vi "Firmware.vi"() -> ()   [LabVIEW 2017]
uses:
  <vilib>/Platform/TimedLoop/XDataNode/timing_clust.ctl
  <vilib>/Platform/TimedLoop/XDataNode/nitl_modes.ctl
  <vilib>/Platform/TimedLoop/XDataNode/wakeup.ctl
  <vilib>/NI/PowerElectronicsControl/Buck-Boost/FPGA/modInput.ctl
  <vilib>/NI/PowerElectronicsControl/ActiveFrontEnd/AFE/Inputs.ctl
  <instrlib>/_niInstr/Instruction Framework/v1/FPGA/Helper Classes/Single Address Space Collection/Single Address Space Collection.lvclass
  C:/Program Files (x86)/National Instruments/LabVIEW 2017/instr.lib/_niInstr/Instruction Framework/v1/FPGA/Interfaces/Address Space Collection/Address Space Collection.lvclass
  <instrlib>/_niInstr/FIFO Register Bus/v1/FPGA/niInstr FIFO Register Bus v1 FPGA.lvclass
  C:/Program Files (x86)/National Instruments/LabVIEW 2017/instr.lib/_niInstr/Instruction Framework/v1/FPGA/Interfaces/Instruction Producer/Instruction Producer.lvclass
  <vilib>/rvi/Emulation/niFpgaGetClockAttributes.vi
  <vilib>/rvi/Emulation/niFpgaSctlEmulationGetInTimedLoop.vi
  <vilib>/rvi/Emulation/niFpgaEmulationReportErrorSimple.vi
  <vilib>/rvi/Emulation/niFpgaProcessEmulError.vi
  <vilib>/rvi/Emulation/niFpgaCriticalErrorInLSC.vi
  <vilib>/rvi/eio/common/nirviEmuTemplateMethod_errors.vi
  <vilib>/rvi/Emulation/niFpgaEmulationIsFPGAContextNoSignature.vi
  <vilib>/rvi/DataTransferAndStorage/Container/Common/niFpgaContainerGetUniqueNameForEmu.vi
  <vilib>/rvi/Memory/Memory_Emulation/niFpgaMemoryEmulationCacheClearOnFirstRun.vi
  <vilib>/rvi/Memory/Memory_Emulation/nirvimemoryEmulationManagerCache_MakeExclusive.vi
  <vilib>/rvi/Memory/Memory_Emulation/niFpgaMemoryEmulationValidateCache.vi
  <vilib>/rvi/Memory/Memory_Emulation/nirvimemoryEmulationManagerCache_InsertValue.vi
  <vilib>/Utility/error.llb/Clear Errors.vi
  <vilib>/rvi/Memory/Memory_Emulation/nirvimemoryEmulationManagerCache_ReleaseExclusive.vi
  <vilib>/rvi/Memory/Memory_Emulation/nirvimemoryEmulationManagerCache_GetValue.vi
  <vilib>/rvi/Memory/Memory_Emulation/nirvimemoryEmulationManagerCache_SetValue.vi
  <userlib>/_NI FLP Library/addons/PowerElectronics/ABCtoAlphaBeta_3PhaseUnitaryMagnitude/FlpLib ABCtoAlphaBeta_3PhaseUnitaryMagnitude 1.vi
  <userlib>/_NI FLP Library/FPGA/outsideSCTL/FlpLib Sine & Cosine Shared Instance 1.vi
  <userlib>/_NI FLP Library/addons/PowerElectronics/AlphaBetaToDQ_noSine/FlpLib AlphaBetaToDQ_noSine 1.vi
  <vilib>/rvi/DataTransferAndStorage/Container/Common/niFpgaContainerExecOnDevCompGetState.vi
  <userlib>/_NI FLP Library/addons/PowerElectronics/SpaceVectorPWM/FlpLib SpaceVectorPWM 2.vi
  <vilib>/rvi/DataTransferAndStorage/Container/Common/niFpgaContainerSetEmuInfo.vi
  <vilib>/rvi/eio/common/nirviEmuReportErrorAndStop.vi
  <vilib>/eio/EIONode/EIONode.xnode
  <vilib>/Platform/TimedLoop/XDataNode/XDataNode.xnode
  <vilib>/rvi/DataTransferAndStorage/Container/XNode/niFpgaContainer.xnode
  <vilib>/rvi/DataTransferAndStorage/Register/Emulation/niFpgaRegisterEmulation.vi
  <vilib>/rvi/DataTransferAndStorage/Register/Emulation/niFpgaRegisterEmulationRefIn.vi
  <vilib>/rvi/LocalResourceManager/LocalResourceManager.xnode
  <instrlib>/_niInstr/Instruction Framework/v1/FPGA/Top Level Bus/Register Configuration/Register Configuration.lvclass
  <vilib>/Platform/TimedLoop/XDataNode/XDNodeRunTimeDep.lvlib
  <vilib>/NI/PowerElectronicsControl/ScaleAndLimit/Core/ScaleAndLimit.lvlib
  <vilib>/NI/PowerElectronicsControl/ScaleAndLimit/Core/AddressSpace.lvclass
  <vilib>/NI/PowerElectronicsControl/WaveformAcq/FPGA/WaveformAddressSpace.lvclass
  <vilib>/NI/PowerElectronicsControl/Buck-Boost/FPGA/BuckBoost.lvlib
  <vilib>/NI/PowerElectronicsControl/Buck-Boost/FPGA/AddressSpace.lvclass
  <vilib>/NI/PowerElectronicsControl/ActiveFrontEnd/AFE/ActiveFrontEnd.lvlib
  <vilib>/NI/PowerElectronicsControl/ActiveFrontEnd/AFE/AddressSpace.lvclass
  <vilib>/NI/PowerElectronicsControl/SVPWM/SVPWM/AddressSpace.lvclass
  <vilib>/NI/PowerElectronicsControl/SVPWM/SVPWM/SVPWM.lvlib
  <vilib>/NI/PowerElectronicsControl/ThreePhasePLL/FPGA/ThreePhasePLL.lvlib
  <vilib>/NI/PowerElectronicsControl/ThreePhasePLL/FPGA/AddressSpace.lvclass
panel:
  out "Vw_AFE":sgl
  out "Vv_AFE":sgl
  out "Vu_AFE":sgl
  out "VLoad":sgl
  out "VDCLink":sgl
  out "gridFrequency":sgl
  in  "PrechargeBuckBoost":bool
  in  "PrechargeAFE":bool
  in  "MainContactor":bool
  in  "ConnectDCLinks":bool
  in  "enableAFE":bool
  in  "I_setpt":sgl format="%#_13g"
  out "I_BuckBoost":sgl[](array[numeric])
  in  "desiredBuckBoostRate":u32
  out "actualBuckBoostRate":u32
  out "FaultBuffer":u64 format="%.0x"
  out "LimitsFlag":bool
  out "Sourcing_P1_DI":u16
  out "Sourcing_P0_DI":u16
  out "Sinking_DO":u32 format="%.0x"
  out "Scanned_AI":sgl[](array[numeric])
  out "AO":i16[](array[numeric])
  out "RelayControl_DO":u8 format="%.0x"
  out "LVTTL_DIO":u32 format="%.0x"
  out "HalfBridge":u16 format="%.0x"
  out "TriggerTimestamp":i32
  out "relativeTimestamp":i32
  in  "ManualTrigger":bool
  in  "fifo reg bus ctrl 0":u32
  out "fifo reg bus status 0":u32
  out "fifo reg bus data 0":u64
  out "SimultaneousAILoopRate":u32
  out "Simultaneous_AI":sgl[](array[numeric])
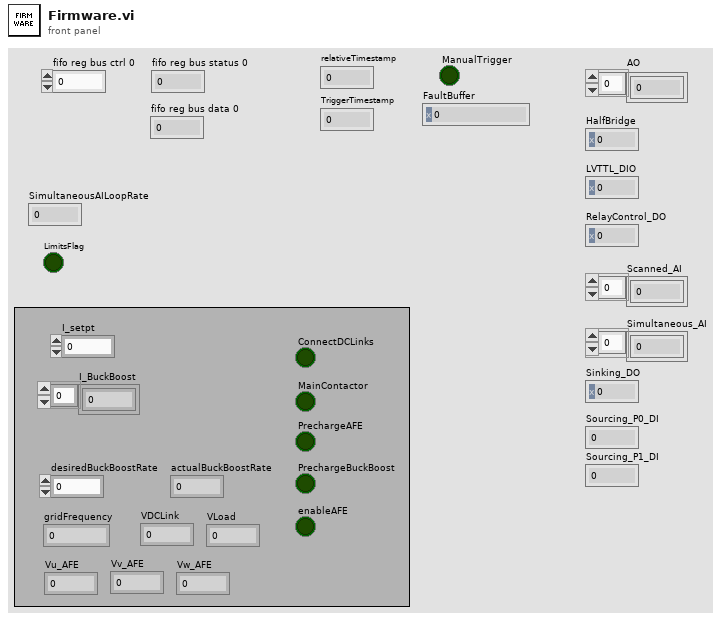
[diagram p1: front panel]
types:
  T1 = typedef "SVPWM.lvlib/Parameters.ctl" = cluster{"Deadtime":refnum<k21>, "Period":refnum<k21>, "A_timing":refnum<k21>, "B_timing":refnum<k21>, "C_timing":refnum<k21>}
  T2 = typedef "BuckBoost.lvlib/contSettings.ctl" = cluster{"numberOfInterleaves":refnum<k21>, "rampRate":refnum<k21>, "manualInput":refnum<k21>, "perturbAmp":refnum<k21>, "perturbAngleInc":refnum<k21>, "reset":refnum<k21>, "state":refnum<k21>, "gains":refnum<k21>, "Currents":refnum<k21>}
  T3 = typedef "BuckBoost.lvlib/modRegisters.ctl" = cluster{"numberOfInterleaves":refnum<k21>, "Enable":refnum<k21>, "triangleInc":refnum<k21>, "Deadband":refnum<k21>, "Enabled":refnum<k21>}
  T4 = typedef "ActiveFrontEnd.lvlib/ControllerRegisters.ctl" = cluster{"Parameters":refnum<k21>, "VDCLinkToP_PISettings":refnum<k21>, "ID_to_VD_PISettings":refnum<k21>, "IQ_to_VQ_PISettings":refnum<k21>, "VDCLink":refnum<k21>, "P":refnum<k21>, "Q":refnum<k21>, "pf":refnum<k21>}
  T5 = typedef "ThreePhasePLL.lvlib/registers.ctl" = cluster{"PLLGains":refnum<k21>, "PLLRange":refnum<k21>, "PLL_reset":refnum<k21>, "PLL_locked":refnum<k21>, "freqBoundaries":refnum<k21>, "expectedFreq":refnum<k21>, "lockDuration":refnum<k21>, "dT":refnum<k21>, "detectedFreq":refnum<k21>, "adjustTheta":refnum<k21>, "HarmonicFilter":refnum<k21>, "HarmonicFilterEnable":refnum<k21>}
  T6 = typedef "XDNodeRunTimeDep.lvlib/timing_clust.ctl" = cluster{"Expected End [f-1]":u64, "Actual End [f-1]":u64, "Finished Late? [f-1]":bool, "Expected End [i-1]":u64, "Actual End [i-1]":u64, "Finished Late? [i-1]":bool, "Expected Start [i]":u64, "Actual Start [i]":u64, "Expected Start [f]":u64, "Actual Start [f]":u64, "Source Name":string, "Structure Name":string, "Period":i64, "Deadline":i64, "Offset":i64, "Start":i64, "Priority":i32, "Timeout":i32, "Mode":T7, "Wakeup Reason":T8, "Error":errorcluster, "Source Type":string, "Secondary Source Type":string, "Global End Time":u64, "Global Start Time":u64, "Frame Duration":u64, "Iteration Duration":u64, "Assigned CPU":i32, "I/O Scan Engine Mode":u32}
  T7 = typedef "XDNodeRunTimeDep.lvlib/nitl_modes.ctl" = enum32{"No Change", "Process missed periods, maintain original phase", "Discard missed periods, maintain original phase", "Process missed periods, ignore original phase", "Discard missed periods, ignore original phase"}
  T8 = typedef "XDNodeRunTimeDep.lvlib/wakeup.ctl" = enum32{"Normal", "Aborted", "Asynchronous wakeup", "Timing source error", "Timed loop error", "Timeout"}
  T9 = typedef "ActiveFrontEnd.lvlib/Inputs.ctl" = cluster{"VgridD":sgl, "VgridQ":sgl, "IgridD":sgl, "IgridQ":sgl, "VDCLink":sgl, "sinTheta":sgl, "cosTheta":sgl}
  T10 = typedef "BuckBoost.lvlib/modInput.ctl" = cluster{"signal":fxp<+,18,0>[]}
  T11 = typedef "niFpgaPID_PIState.ctl" = cluster{"uI(k-1)":sgl, "e(k-1)":sgl, "output (k-1)":sgl}
  T12 = cluster{"PIstateOut":T11, "filter0":sgl, "filter1":sgl}
  T13 = typedef "ActiveFrontEnd.lvlib/Outputs.ctl" = cluster{"VcmdAlpha":sgl, "VcmdBeta":sgl, "VcmdD":sgl, "VcmdQ":sgl, "IcmdD":sgl, "IcmdQ":sgl, "P":sgl, "Q":sgl, "Pf":sgl, "perturbance":sgl}
  T14 = typedef "ON_OFF.ctl" = cluster{"ON":u32, "OFF":u32}
  T15 = typedef "ScaleAndLimit.lvlib/LimitsRegisters.ctl" = cluster{"HighLimits":refnum<k21>, "LowLimits":refnum<k21>, "ClearLimits":refnum<k21>, "LimitsFlag":refnum<k21>}
  T16 = typedef "ScaleAndLimit.lvlib/ConfigRegisters.ctl" = cluster{"LimitsEnabled":refnum<k21>, "UnscaledHighLimit":refnum<k21>, "UnscaledLowLimit":refnum<k21>, "B":refnum<k21>, "M":refnum<k21>}
  T17 = typedef "BuckBoost.lvlib/modOutput.ctl" = cluster{"Top":bool, "Bottom":bool}
  T18 = typedef "SVPWM.lvlib/SwitchPositions.ctl" = cluster{"A_Top":bool, "A_Bot":bool, "B_Top":bool, "B_Bot":bool, "C_Top":bool, "C_Bot":bool}
  T19 = cluster{"VcmdAlpha":sgl, "VcmdBeta":sgl, "VcmdD":sgl, "VcmdQ":sgl, "IcmdD":sgl, "IcmdQ":sgl, "P":sgl, "Q":sgl, "Pf":sgl, "perturbance":sgl}
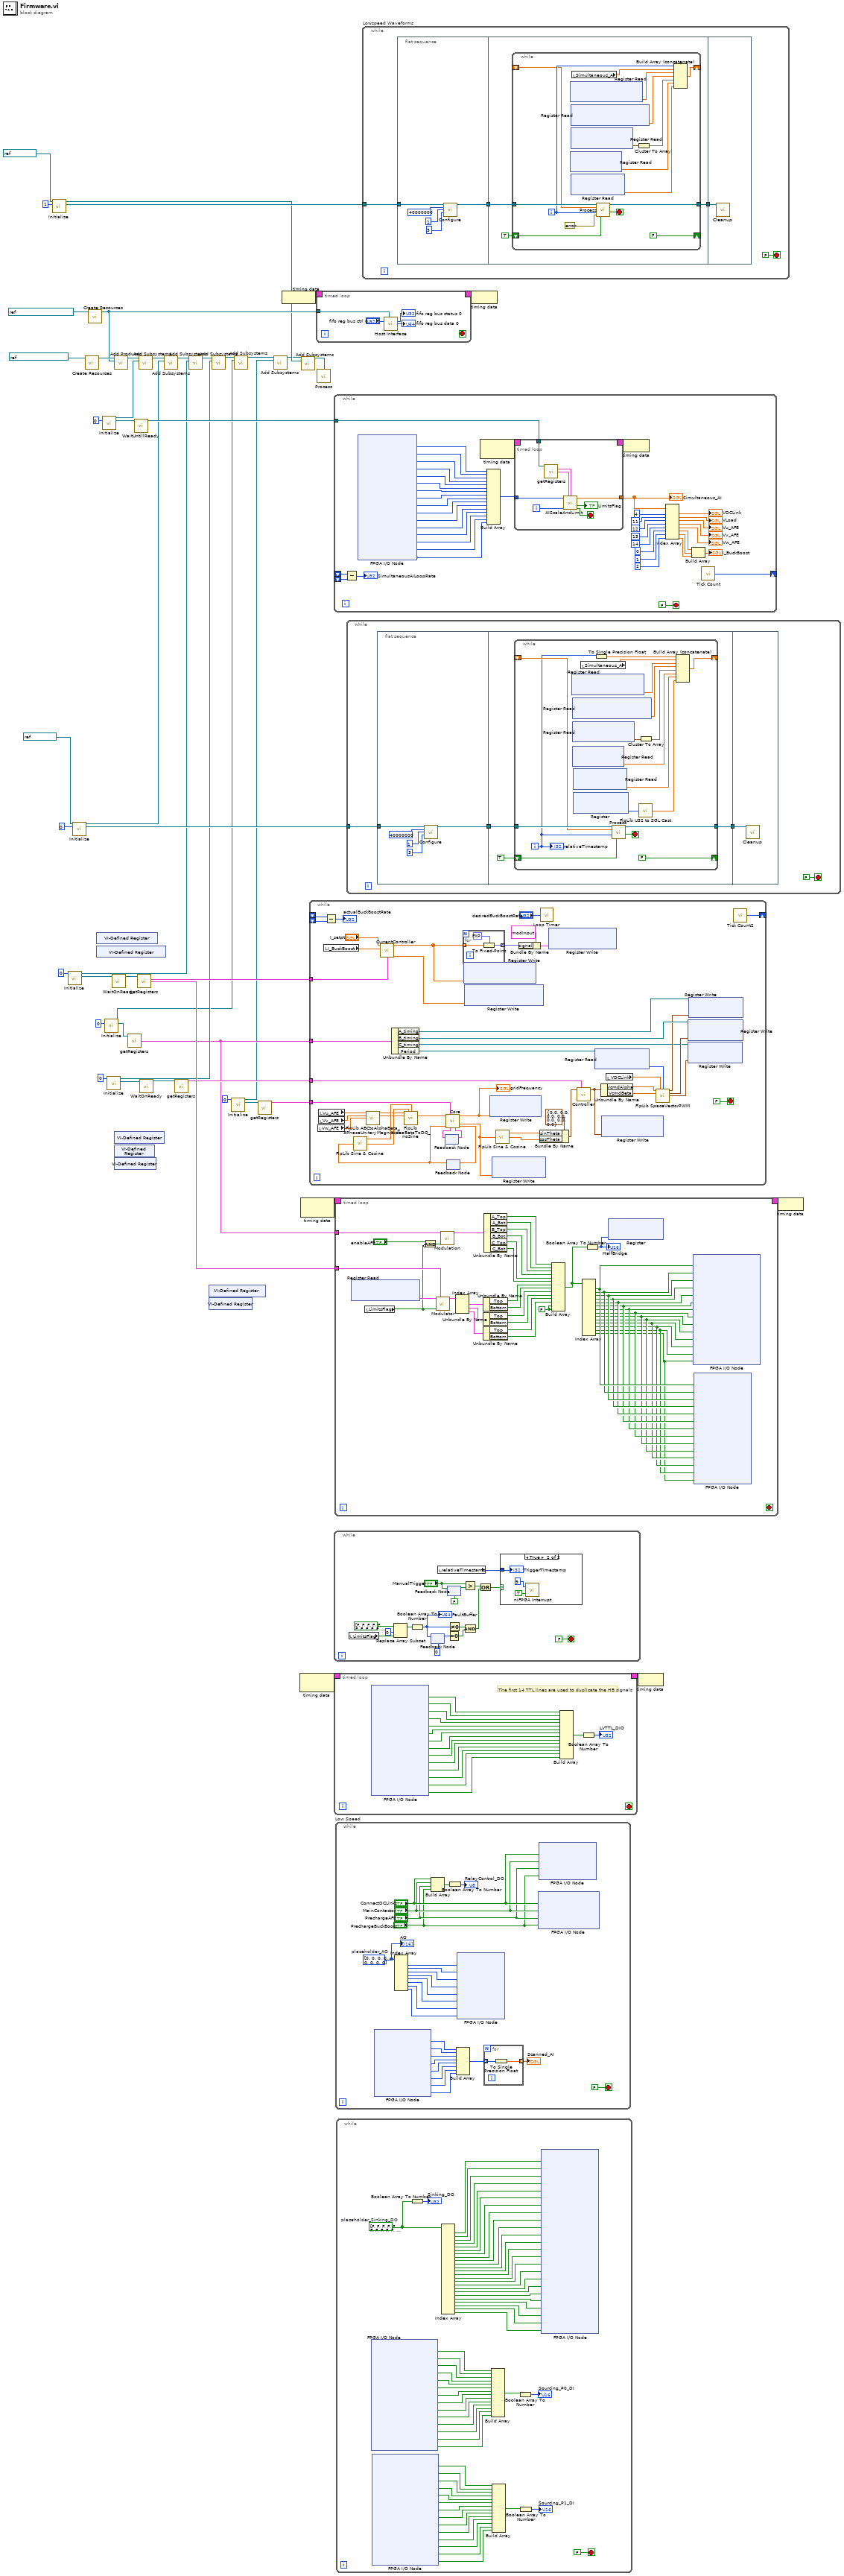
[diagram p0: block diagram]
diagram:
  n1 = call <vilib>:"Initialize.vi"("DMA FIFO"=refnum<k21> "DataSGL1" ("FIFO Out"), "instance"=u8 1) -> ("subsystem"=w28:refnum<class "Single Address Space Collection.lvclass">, "AddressSpace"=w31:refnum<class "WaveformAddressSpace.lvclass">)  [unwired: 12 in]
  n2 = call <vilib>:"Initialize.vi"("instance"=u8 0) -> ("subsystem"=w18:refnum<class "Single Address Space Collection.lvclass">, "AddressSpace"=w24:refnum<class "AddressSpace.lvclass">)  [unwired: 13 in]
  n3 = call <vilib>:"Initialize.vi"("DMA FIFO"=refnum<k21> "DataSGL0" ("FIFO Out"), "instance"=u8 0) -> ("subsystem"=w34:refnum<class "Single Address Space Collection.lvclass">, "AddressSpace"=w36:refnum<class "WaveformAddressSpace.lvclass">)  [unwired: 12 in]
  n4 = call <instrlib>:"Create Resources.vi"("register clock"=refnum<k21> "40 MHz Onboard Clock") -> ("register configuration"=w47:refnum<class "Register Configuration.lvclass">)  [unwired: 14 in]
  n5 = call <instrlib>:"Create Resources.vi"("instruction fifo"=refnum<k21> "reg.host instruction fifo 0") -> ("fifo register bus"=w39:refnum<class "niInstr FIFO Register Bus v1 FPGA.lvclass">)  [unwired: 14 in]
  n6 = xnode "VI-Defined Register"() -> ()  [unwired: 1 out]
  n7 = xnode "VI-Defined Register"() -> ()  [unwired: 1 out]
  n8 = call <vilib>:"Initialize.vi"("instance"=u8 0) -> ("subsystem"=w44:refnum<class "Single Address Space Collection.lvclass">, "AddressSpace"=w42:refnum<class "AddressSpace.lvclass">)  [unwired: 13 in]
  n9 = call <vilib>:"Initialize.vi"("instance"=u8 0) -> ("subsystem"=w8:refnum<class "Single Address Space Collection.lvclass">, "AddressSpace"=w10:refnum<class "AddressSpace.lvclass">)  [unwired: 13 in]
  n10 = call <vilib>:"Initialize.vi"("instance"=u8 0) -> ("subsysytem"=w12:refnum<class "Single Address Space Collection.lvclass">, "AddressSpace"=w16:refnum<class "AddressSpace.lvclass">)  [unwired: 13 in]
  n11 = call <vilib>:"WaitOnReady.vi"("AddressSpace in"=w24) -> ("AddressSpace out"=w23:refnum<class "AddressSpace.lvclass">)  [unwired: 14 in]
  n12 = xnode "VI-Defined Register"() -> ()  [unwired: 1 out]
  n13 = call <instrlib>:"Add Producer.vi"("register configuration in"=w47, "instruction producer"=w39) -> ("register configuration out"=w45:refnum<class "Register Configuration.lvclass">)  [unwired: 13 in]
  n14 = xnode "VI-Defined Register"() -> ()  [unwired: 1 out]
  n15 = xnode "VI-Defined Register"() -> ()  [unwired: 1 out]
  n16 = call <vilib>:"getRegisters.vi"("AddressSpace in"=w10) -> ("Parameters"=w7:T1)  [unwired: 13 in, 1 out]
  n17 = call <vilib>:"WaitUntillReady.vi"("AddressSpace in"=w42) -> ("AddressSpace out"=w41:refnum<class "AddressSpace.lvclass">)  [unwired: 14 in]
  n18 = call <vilib>:"getRegisters.vi"("AddressSpace in"=w23) -> ("settingsReg"=w22:T2, "modRegisters"=w21:T3)  [unwired: 12 in, 1 out]
  n19 = call <instrlib>:"Add Subsystems.vi"("register configuration in"=w45, "subsystems"=w44) -> ("register configuration out"=w35:refnum<class "Register Configuration.lvclass">)  [unwired: 13 in]
  n20 = call <vilib>:"WaitOnReady.vi"("AddressSpace in"=w16) -> ("AddressSpace out"=w15:refnum<class "AddressSpace.lvclass">)  [unwired: 14 in]
  n21 = call <instrlib>:"Add Subsystems.vi"("register configuration in"=w35, "subsystems"=w34) -> ("register configuration out"=w19:refnum<class "Register Configuration.lvclass">)  [unwired: 13 in]
  n22 = call <vilib>:"getRegisters.vi"("AddressSpace in"=w15) -> ("CntlRegisters"=w14:T4)  [unwired: 14 in]
  n23 = call <instrlib>:"Add Subsystems.vi"("register configuration in"=w19, "subsystems"=w18) -> ("register configuration out"=w13:refnum<class "Register Configuration.lvclass">)  [unwired: 13 in]
  n24 = xnode "VI-Defined Register"() -> ()  [unwired: 1 out]
  n25 = xnode "VI-Defined Register"() -> ()  [unwired: 1 out]
  n26 = call <instrlib>:"Add Subsystems.vi"("register configuration in"=w13, "subsystems"=w12) -> ("register configuration out"=w9:refnum<class "Register Configuration.lvclass">)  [unwired: 13 in]
  n27 = call <vilib>:"Initialize.vi"("instance"=u8 0) -> ("subsysytem"=w2:refnum<class "Single Address Space Collection.lvclass">, "AddressSpace"=w6:refnum<class "AddressSpace.lvclass">)  [unwired: 13 in]
  n28 = call <instrlib>:"Add Subsystems.vi"("register configuration in"=w9, "subsystems"=w8) -> ("register configuration out"=w4:refnum<class "Register Configuration.lvclass">)  [unwired: 13 in]
  n29 = call <vilib>:"getRegisters.vi"("AddressSpace"=w6) -> ("registers"=w1:T5)  [unwired: 14 in]
  n30 = call <instrlib>:"Add Subsystems.vi"("register configuration in"=w4, "subsystems"=w2) -> ("register configuration out"=w3:refnum<class "Register Configuration.lvclass">)  [unwired: 13 in]
  n31 = node-c288() -> (w49:T6)
  n32 = node-c288() -> (w33:T6)  [unwired: 1 in]
  n33 = node-c288() -> (w26:T6)  [unwired: 1 in]
  n34 = call <instrlib>:"Add Subsystems.vi"("register configuration in"=w3, "subsystems"=w28) -> ("register configuration out"=w27:refnum<class "Register Configuration.lvclass">)  [unwired: 13 in]
  n35 = while {
    shift-right: [w94] -> _
    shift-left: _ -> [w92]
    shift-left: _ -> [w93]
    tunnel: w22 -> [w89]
    tunnel: w14 -> [w83]
    tunnel: w7 -> [w82]
    tunnel: w1 -> [w66]
    stop <- FALSE stop-if-true
    n36 = local read "Vw_AFE"() -> (w55:sgl)
    n37 = local read "Vu_AFE"() -> (w57:sgl)
    n38 = local read "Vv_AFE"() -> (w56:sgl)
    n39 = local read "I_BuckBoost"() -> (w50:sgl[])
    n40 = Subtract(x=w92, y=w93) -> (x-y=→"actualBuckBoostRate":u32)
    n41 = call-poly <userlib>:"FlpLib ABCtoAlphaBeta_3PhaseUnitaryMagnitude.vi"("A"=w57, "B"=w56, "C"=w55) -> ("alpha"=w68:sgl, "beta"=w69:sgl)  [unwired: 11 in]
    n42 = call <vilib>:"CurrentController.vi"("I_setpt"="I_setpt", "I_procVar"=w50, "settings"=w89) -> ("output"=w60:sgl[], "perturbance"=w59:sgl)  [unwired: 11 in]
    n43 = Unbundle By Name(w82) -> ("A_timing"=w79:refnum<k21>, "B_timing"=w78:refnum<k21>, "C_timing"=w75:refnum<k21>, "Period"=w81:refnum<k21>)
    n44 = feedback #1() -> (w51:T12)  [unwired: 1 in]
    n45 = feedback #2() -> (w73:sgl)  [unwired: 1 in]
    n46 = call-poly <userlib>:"FlpLib Sine & Cosine.vi"("x"=w73) -> ("cos(x)"=w70:sgl, "sin(x)"=w71:sgl)  [unwired: 3 in]
    n47 = call-poly <userlib>:"FlpLib AlphaBetaToDQ_noSine.vi"("alpha"=w68, "cosx"=w70, "sinx"=w71, "beta"=w69) -> ("quadrature"=w72:sgl)  [unwired: 10 in, 1 out]
    n48 = call <vilib>:"Core.vi"("Vq"=w72, "registers"=w66, "ThetaIn"=w73, "StateIn"=w51) -> ("gridFrequency"=w54:sgl, "adjustedTheta"=w53:sgl, "StateOut"=w52:T12, "ThetaOut"=w67:sgl)  [unwired: 7 in, 1 out]
    "gridFrequency" <- w54
    n49 = feedback-in #1(w52) -> ()
    n50 = feedback-in #2(w67) -> ()
    n51 = for {
      tunnel: w60 -> [w97] mode=indexing
      tunnel: [w98] -> w87 mode=indexing
      n52 = To Fixed-Point(fixed-point type=fxp<+,18,0> 0.0 ("triangle"), number=w97) -> (fixed-point=w98:fxp<+,18,0>)
    }
    n53 = xnode ("Register Write")("Data"=w60) -> ()  [unwired: 1 in, 1 out]
    n54 = xnode ("Register Write")("Data"=w59) -> ()  [unwired: 1 in, 1 out]
    n55 = xnode ("Register Write")("Data"=w54) -> ()  [unwired: 1 in, 1 out]
    n56 = xnode ("Register Write")("Data"=w53) -> ()  [unwired: 1 in, 1 out]
    n57 = call-poly <userlib>:"FlpLib Sine & Cosine.vi"("x"=w53) -> ("cos(x)"=w63:sgl, "sin(x)"=w64:sgl)  [unwired: 3 in]
    n58 = Bundle By Name(cluster=T10 {"signal"=[0.0, 0.0, 0.0, 0.0]} ("input"), "signal"=w87) -> (w86:T10)
    n59 = Bundle By Name(cluster=T9 {"VgridD"=0.0, "VgridQ"=0.0, "IgridD"=0.0, "IgridQ"=0.0, "VDCLink"=0.0, "sinTheta"=0.0, "cosTheta"=0.0} ("Inputs"), "sinTheta"=w64, "cosTheta"=w63) -> (w62:T9)
    n60 = call "Loop Timer"("Count(Ticks)"="desiredBuckBoostRate") -> ()  [unwired: 1 out]
    n61 = xnode ("Register Write")("Data"=w86) -> ()  [unwired: 1 in, 1 out]
    n62 = call <vilib>:"Controller.vi"("Inputs"=w62, "Registers"=w83) -> ("Outputs"=w61:T13)  [unwired: 13 in]
    n63 = xnode ("Register Read")("Register In"=w81) -> ("Data"=w80:u32)  [unwired: 1 out]
    n64 = Unbundle By Name(w61) -> ("VcmdAlpha"=w84:sgl, "VcmdBeta"=w85:sgl)
    n65 = xnode ("Register Write")("Data"=w61) -> ()  [unwired: 1 in, 1 out]
    n66 = local read "VDCLink"() -> (w58:sgl)
    n67 = call-poly <userlib>:"FlpLib SpaceVectorPWM.vi"("ref_alpha"=w84, "ref_max"=w58, "Period"=w80, "ref_beta"=w85) -> ("A"=w77:T14, "B"=w76:T14, "C"=w74:T14)  [unwired: 8 in, 1 out]
    n68 = xnode ("Register Write")("Data"=w74, "Register In"=w75) -> ()  [unwired: 1 out]
    n69 = xnode ("Register Write")("Data"=w76, "Register In"=w78) -> ()  [unwired: 1 out]
    n70 = xnode ("Register Write")("Data"=w77, "Register In"=w79) -> ()  [unwired: 1 out]
    n71 = call "Tick Count2"() -> ("Tick Count(Ticks)"=w94:u32)
  }
  n72 = timed-loop {
    timing: w49 -> [_]
    timing-out: [_] -> w48
    tunnel: w39 -> [w103]
    stop <- _ stop-if-true
    n73 = call <instrlib>:"Host Interface.vi"("fifo register bus"=w103, "fifo reg bus ctrl 0"="fifo reg bus ctrl 0") -> ("fifo reg bus status 0"=→"fifo reg bus status 0":u32, "fifo reg bus data 0"=→"fifo reg bus data 0":u64)  [unwired: 12 in]
  }
  n74 = call <instrlib>:"Process.vi"("register configuration"=w27) -> ()  [unwired: 15 in]
  n75 = while {
    shift-right: [w147] -> _
    shift-left: _ -> [w146]
    shift-left: _ -> [w145]
    tunnel: w41 -> [w135]
    stop <- FALSE stop-if-true
    n76 = Subtract(x=w146, y=w145) -> (x-y=→"SimultaneousAILoopRate":u32)
    n77 = xnode "FPGA I/O Node"() -> ("I0_BuckBoost"=w143:i16, "I1_BuckBoost"=w142:i16, "I2_BuckBoost"=w141:i16, "Vgrid_BuckBoost"=w140:i16, "VDCLink_BuckBoost"=w139:i16, "V0_BuckBoost"=w138:i16, "V1_BuckBoost"=w133:i16, "V2_BuckBoost"=w132:i16, "Iu_AFE"=w131:i16, "Iv_AFE"=w130:i16, "Iw_AFE"=w129:i16, "VLoad_BuckBoost"=w128:i16, "Vu_AFE"=w127:i16, "Vv_AFE"=w126:i16, "Vw_AFE"=w125:i16, "VDCLink_AFE"=w124:i16)  [unwired: 16 in, 16 out]
    n78 = node-c288() -> (w137:T6)  [unwired: 1 in]
    n79 = Build Array(w143, w142, w141, w140, w139, w138, w133, w132, w131, w130, w129, w128, w127, w126, w125, w124) -> (w134:i16[])
    n80 = timed-loop {
      timing: w137 -> [_]
      timing-out: [_] -> w136
      tunnel: w134 -> [w156]
      tunnel: [w155] -> w123
      tunnel: w135 -> [w153]
      i -> [w150]
      stop <- w154 stop-if-true
      n81 = call <vilib>:"getRegisters.vi"("AddressSpace in"=w153) -> ("LimitsRegisters"=w151:T15, "ConfigRegisters"=w152:T16)  [unwired: 12 in, 1 out]
      n82 = call <vilib>:"AIScaleAndLimit.vi"("UnscaledAI"=w156, "ConfigRegisters"=w152, "LimitsRegisters"=w151, "index"=w150) -> ("ScaledAI"=w155:sgl[], "Limited"=→"LimitsFlag":bool, "output valid"=w154:bool)  [unwired: 9 in]
    }
    "Simultaneous_AI" <- w123
    n83 = node-c288(w136) -> ()
    n84 = Index Array(array=w123, index #1=4 ("index"), index #2=11 ("index"), index #3=12 ("index"), index #4=13 ("index"), index #5=14 ("index"), index #6=0 ("index"), index #7=1 ("index"), index #8=2 ("index")) -> (element #1=→"VDCLink":sgl, element #2=→"VLoad":sgl, element #3=→"Vu_AFE":sgl, element #4=→"Vv_AFE":sgl, element #5=→"Vw_AFE":sgl, element #6=w109:sgl, element #7=w108:sgl, element #8=w107:sgl)
    n85 = Build Array(w109, w108, w107) -> (→"I_BuckBoost":sgl[])
    n86 = call "Tick Count"() -> ("Tick Count(Ticks)"=w147:u32)
  }
  n87 = while {
    stop <- FALSE stop-if-true
    n88 = local read "LimitsFlag"() -> (w169:bool)
    n89 = Replace Array Subset(array=bool[] [FALSE, FALSE, FALSE, FALSE, FALSE, FALSE, FALSE, FALSE, FALSE, FALSE, FALSE, FALSE, FALSE, FALSE, FALSE, FALSE, FALSE, FALSE, FALSE, FALSE, FALSE, FALSE, FALSE, FALSE, FALSE, FALSE, FALSE, FALSE, FALSE, FALSE, FALSE, FALSE, FALSE, FALSE, FALSE, FALSE, FALSE, FALSE, FALSE, FALSE, FALSE, FALSE, FALSE, FALSE, FALSE, FALSE, FALSE, FALSE, FALSE, FALSE, FALSE, FALSE, FALSE, FALSE, FALSE, FALSE, FALSE, FALSE, FALSE, FALSE, FALSE, FALSE, FALSE, FALSE], new element=w169, index=0) -> (w167:bool[])
    n90 = Boolean Array To Number(Boolean array=w167) -> (number=w165:u64)
    "FaultBuffer" <- w165
    n91 = feedback-in #3(w165) -> ()
    n92 = feedback #3(u64 0) -> (w164:u64)
    n93 = local read "relativeTimestamp"() -> (w171:i32)
    n94 = feedback-in #4("ManualTrigger") -> ()
    n95 = feedback #4(FALSE ("ManualTrigger")) -> (w175:bool)
    n96 = Equal To 0?(x=w164) -> (x = 0?=w162:bool)
    n97 = Not Equal To 0?(x=w165) -> (x != 0?=w163:bool)
    n98 = Greater?(x="ManualTrigger", y=w175) -> (0:w176:bool)
    n99 = Compound Arithmetic op=AND(w163, w162) -> (w161:bool)
    n100 = Compound Arithmetic op=OR(w176, w161) -> (w173:bool)
    n101 = case shown="True" w173 {
      tunnel: w171 -> [_ w178]
      frame False {
      }
      frame True {
        n102 = call <vilib>:"niFPGA Interrupt.vi"("Wait Until Cleared (F)"=TRUE, "IRQ Number (0)"=u8 9) -> ()  [unwired: 1 in]
        "TriggerTimestamp" <- w178
      }
    }
  }
  n103 = timed-loop {
    timing: w33 -> [_]
    timing-out: [_] -> w32
    stop <- _ stop-if-true
    # "The first 14 TTL lines are used to duplicate the HB signals"
    n104 = xnode "FPGA I/O Node"() -> ("RMC/LVTTL/DIO18"=w196:bool, "RMC/LVTTL/DIO19"=w195:bool, "RMC/LVTTL/DIO20"=w194:bool, "RMC/LVTTL/DIO21"=w193:bool, "RMC/LVTTL/DIO22"=w192:bool, "RMC/LVTTL/DIO23"=w191:bool, "RMC/LVTTL/DIO24"=w190:bool, "RMC/LVTTL/DIO25"=w189:bool, "RMC/LVTTL/DIO26"=w188:bool, "RMC/LVTTL/DIO27"=w187:bool, "RMC/LVTTL/DIO28"=w186:bool, "RMC/LVTTL/DIO29"=w185:bool, "RMC/LVTTL/DIO30"=w184:bool, "RMC/LVTTL/DIO31"=w183:bool)  [unwired: 14 in, 14 out]
    n105 = Build Array(w196, w195, w194, w193, w192, w191, w190, w189, w188, w187, w186, w185, w184, w183) -> (w182:bool[])
    n106 = Boolean Array To Number(Boolean array=w182) -> (number=→"LVTTL_DIO":u16)
  }
  n107 = timed-loop {
    timing: w26 -> [_]
    timing-out: [_] -> w25
    tunnel: w21 -> [w238]
    tunnel: w7 -> [w236]
    stop <- _ stop-if-true
    w200 = FALSE ("element")
    n108 = xnode ("Register Read")() -> ("Data"=w237:cluster{"signal":fxp<+,18,0>[]})  [unwired: 1 in, 1 out]
    n109 = local read "LimitsFlag"() -> (w234:bool)
    n110 = Compound Arithmetic op=AND("enableAFE", invert w234) -> (w233:bool)
    n111 = call <vilib>:"Modulator.vi"("input"=w237, "modRegisters"=w238, "Disable"=w234) -> ("output"=w232:T17[])  [unwired: 12 in]
    n112 = call <vilib>:"Modulation.vi"("Parameters"=w236, "enable"=w233) -> ("SwitchPositions"=w228:T18)  [unwired: 13 in]
    n113 = Index Array(array=w232) -> (element #1=w231:T17, element #2=w230:T17, element #3=w229:T17)  [unwired: 3 in]
    n114 = Unbundle By Name(w231) -> ("Top"=w221:bool, "Bottom"=w220:bool)
    n115 = Unbundle By Name(w230) -> ("Top"=w219:bool, "Bottom"=w218:bool)
    n116 = Unbundle By Name(w229) -> ("Top"=w217:bool, "Bottom"=w216:bool)
    n117 = Unbundle By Name(w228) -> ("A_Top"=w227:bool, "A_Bot"=w226:bool, "B_Top"=w225:bool, "B_Bot"=w224:bool, "C_Top"=w223:bool, "C_Bot"=w222:bool)
    n118 = Build Array(w227, w226, w225, w224, w223, w222, w221, w220, w219, w218, w217, w216, w200, w200) -> (w215:bool[])
    n119 = Index Array(array=w215) -> (element #1=w214:bool, element #2=w213:bool, element #3=w212:bool, element #4=w211:bool, element #5=w210:bool, element #6=w209:bool, element #7=w208:bool, element #8=w207:bool, element #9=w206:bool, element #10=w205:bool, element #11=w204:bool, element #12=w203:bool, element #13=w202:bool, element #14=w201:bool)  [unwired: 14 in]
    n120 = Boolean Array To Number(Boolean array=w215) -> (number=w199:u16)
    "HalfBridge" <- w199
    n121 = xnode "Register"("Data"=w199) -> ()  [unwired: 1 in, 1 out]
    n122 = xnode "FPGA I/O Node"("RMC/Half-Bridge/DO0"=w214, "RMC/Half-Bridge/DO1"=w213, "RMC/Half-Bridge/DO2"=w212, "RMC/Half-Bridge/DO3"=w211, "RMC/Half-Bridge/DO4"=w210, "RMC/Half-Bridge/DO5"=w209, "RMC/Half-Bridge/DO6"=w208, "RMC/Half-Bridge/DO7"=w207, "RMC/Half-Bridge/DO8"=w206, "RMC/Half-Bridge/DO9"=w205, "RMC/Half-Bridge/DO10"=w204, "RMC/Half-Bridge/DO11"=w203, "RMC/Half-Bridge/DO12"=w202, "RMC/Half-Bridge/DO13"=w201) -> ()  [unwired: 14 in, 14 out]
    n123 = xnode "FPGA I/O Node"("RMC/LVTTL/DIO0"=w214, "RMC/LVTTL/DIO1"=w213, "RMC/LVTTL/DIO2"=w212, "RMC/LVTTL/DIO3"=w211, "RMC/LVTTL/DIO4"=w210, "RMC/LVTTL/DIO5"=w209, "RMC/LVTTL/DIO6"=w208, "RMC/LVTTL/DIO7"=w207, "RMC/LVTTL/DIO8"=w206, "RMC/LVTTL/DIO9"=w205, "RMC/LVTTL/DIO10"=w204, "RMC/LVTTL/DIO11"=w203, "RMC/LVTTL/DIO12"=w202, "RMC/LVTTL/DIO13"=w201) -> ()  [unwired: 14 in, 14 out]
  }
  n124 = while "Low Speed" {
    stop <- FALSE stop-if-true
    w265 = i16[] [0, 0, 0, 0, 0, 0, 0, 0]  # placeholder_AO
    n125 = xnode "FPGA I/O Node"() -> ("RMC/Scanned/AI0"=w255:i16, "RMC/Scanned/AI1"=w254:i16, "RMC/Scanned/AI2"=w253:i16, "RMC/Scanned/AI3"=w252:i16, "RMC/Scanned/AI4"=w251:i16, "RMC/Scanned/AI5"=w250:i16, "RMC/Scanned/AI6"=w249:i16, "RMC/Scanned/AI7"=w248:i16)  [unwired: 8 in, 8 out]
    n126 = Index Array(array=w265) -> (element #1=w264:i16, element #2=w263:i16, element #3=w262:i16, element #4=w261:i16, element #5=w260:i16, element #6=w259:i16, element #7=w258:i16, element #8=w257:i16)  [unwired: 8 in]
    n127 = Build Array("ConnectDCLinks", "MainContactor", "PrechargeAFE", "PrechargeBuckBoost") -> (w245:bool[])
    n128 = Boolean Array To Number(Boolean array=w245) -> (number=→"RelayControl_DO":u8)
    n129 = Build Array(w255, w254, w253, w252, w251, w250, w249, w248) -> (w247:i16[])
    n130 = xnode "FPGA I/O Node"("RMC/AO/AO0"=w264, "RMC/AO/AO1"=w263, "RMC/AO/AO2"=w262, "RMC/AO/AO3"=w261, "RMC/AO/AO4"=w260, "RMC/AO/AO5"=w259, "RMC/AO/AO6"=w258, "RMC/AO/AO7"=w257) -> ()  [unwired: 8 in, 8 out]
    n131 = for {
      tunnel: w247 -> [w268] mode=indexing
      tunnel: [w267] -> w246 mode=indexing
      n132 = To Single Precision Float(number=w268) -> (single precision float=w267:sgl)
    }
    "Scanned_AI" <- w246
    n133 = xnode "FPGA I/O Node"("ConnectDCLinks"="ConnectDCLinks", "MainContactor"="MainContactor", "PrechargeAFE"="PrechargeAFE", "PrechargeBuckBoost"="PrechargeBuckBoost") -> ()  [unwired: 4 in, 4 out]
    n134 = xnode "FPGA I/O Node"("RMC/LVTTL/DIO14"="ConnectDCLinks", "RMC/LVTTL/DIO15"="MainContactor", "RMC/LVTTL/DIO16"="PrechargeAFE", "RMC/LVTTL/DIO17"="PrechargeBuckBoost") -> ()  [unwired: 4 in, 4 out]
    "AO" <- w265
  }
  n135 = while {
    stop <- FALSE stop-if-true
    w326 = bool[] [FALSE, FALSE, FALSE, FALSE, FALSE, FALSE, FALSE, FALSE, FALSE, FALSE, FALSE, FALSE, FALSE, FALSE, FALSE, FALSE, FALSE, FALSE, FALSE, FALSE, FALSE, FALSE, FALSE, FALSE]  # placeholder_Sinking_DO
    n136 = xnode "FPGA I/O Node"() -> ("RMC/Sourcing P0/DI0"=w300:bool, "RMC/Sourcing P0/DI1"=w299:bool, "RMC/Sourcing P0/DI2"=w298:bool, "RMC/Sourcing P0/DI3"=w297:bool, "RMC/Sourcing P0/DI4"=w296:bool, "RMC/Sourcing P0/DI5"=w295:bool, "RMC/Sourcing P0/DI6"=w294:bool, "RMC/Sourcing P0/DI7"=w293:bool, "RMC/Sourcing P0/DI8"=w292:bool, "RMC/Sourcing P0/DI9"=w291:bool, "RMC/Sourcing P0/DI10"=w290:bool, "RMC/Sourcing P0/DI11"=w289:bool, "RMC/Sourcing P0/DI12"=w288:bool, "RMC/Sourcing P0/DI13"=w287:bool)  [unwired: 14 in, 14 out]
    n137 = xnode "FPGA I/O Node"() -> ("RMC/Sourcing P1/DI0"=w269:bool, "RMC/Sourcing P1/DI1"=w270:bool, "RMC/Sourcing P1/DI2"=w271:bool, "RMC/Sourcing P1/DI3"=w272:bool, "RMC/Sourcing P1/DI4"=w273:bool, "RMC/Sourcing P1/DI5"=w274:bool, "RMC/Sourcing P1/DI6"=w275:bool, "RMC/Sourcing P1/DI7"=w276:bool, "RMC/Sourcing P1/DI8"=w277:bool, "RMC/Sourcing P1/DI9"=w278:bool, "RMC/Sourcing P1/DI10"=w279:bool, "RMC/Sourcing P1/DI11"=w280:bool, "RMC/Sourcing P1/DI12"=w281:bool, "RMC/Sourcing P1/DI13"=w282:bool)  [unwired: 14 in, 14 out]
    n138 = Boolean Array To Number(Boolean array=w326) -> (number=→"Sinking_DO":u32)
    n139 = Index Array(array=w326) -> (element #1=w325:bool, element #2=w324:bool, element #3=w323:bool, element #4=w322:bool, element #5=w321:bool, element #6=w320:bool, element #7=w319:bool, element #8=w318:bool, element #9=w317:bool, element #10=w316:bool, element #11=w315:bool, element #12=w314:bool, element #13=w313:bool, element #14=w312:bool, element #15=w311:bool, element #16=w310:bool, element #17=w309:bool, element #18=w308:bool, element #19=w307:bool, element #20=w306:bool, element #21=w305:bool, element #22=w304:bool, element #23=w303:bool, element #24=w302:bool)  [unwired: 24 in]
    n140 = Build Array(w300, w299, w298, w297, w296, w295, w294, w293, w292, w291, w290, w289, w288, w287) -> (w286:bool[])
    n141 = Build Array(w269, w270, w271, w272, w273, w274, w275, w276, w277, w278, w279, w280, w281, w282) -> (w283:bool[])
    n142 = Boolean Array To Number(Boolean array=w286) -> (number=→"Sourcing_P0_DI":u16)
    n143 = Boolean Array To Number(Boolean array=w283) -> (number=→"Sourcing_P1_DI":u16)
    n144 = xnode "FPGA I/O Node"("RMC/Sinking/DO0"=w325, "RMC/Sinking/DO1"=w324, "RMC/Sinking/DO2"=w323, "RMC/Sinking/DO3"=w322, "RMC/Sinking/DO4"=w321, "RMC/Sinking/DO5"=w320, "RMC/Sinking/DO6"=w319, "RMC/Sinking/DO7"=w318, "RMC/Sinking/DO8"=w317, "RMC/Sinking/DO9"=w316, "RMC/Sinking/DO10"=w315, "RMC/Sinking/DO11"=w314, "RMC/Sinking/DO12"=w313, "RMC/Sinking/DO13"=w312, "RMC/Sinking/DO14"=w311, "RMC/Sinking/DO15"=w310, "RMC/Sinking/DO16"=w309, "RMC/Sinking/DO17"=w308, "RMC/Sinking/DO18"=w307, "RMC/Sinking/DO19"=w306, "RMC/Sinking/DO20"=w305, "RMC/Sinking/DO21"=w304, "RMC/Sinking/DO22"=w303, "RMC/Sinking/DO23"=w302) -> ()  [unwired: 24 in, 24 out]
  }
  n145 = while {
    tunnel: w36 -> [w328]
    stop <- FALSE stop-if-true
    n146 = flat-sequence {
      tunnel: [w332] -> w330
      tunnel: w328 -> [w333]
      tunnel: w330 -> [w339]
      tunnel: [w338] -> w329
      tunnel: w329 -> [w358]
      frame #0 {
        n147 = call <vilib>:"Configure.vi"("WaveformAddressSpace in"=w333, "oclk_freq"=u32 40000000, "oclk_mult"=u32 1, "UnderflowMargin"=u32 3 ("y")) -> ("WaveformAddressSpace out"=w332:refnum<class "WaveformAddressSpace.lvclass">)  [unwired: 11 in]
      }
      frame #1 {
        n148 = while {
          shift-right: [w356] -> _
          shift-left: _ -> [w350]
          shift-right: [FALSE] -> _
          shift-left: TRUE -> [w352]
          tunnel: w339 -> [w354]
          tunnel: [w353] -> w338
          i -> [w349]
          stop <- w355 stop-if-true
          n149 = xnode ("Register Read")() -> ("Data"=w346:sgl[])  [unwired: 1 in, 1 out]
          n150 = xnode ("Register Read")() -> ("Data"=w345:sgl)  [unwired: 1 in, 1 out]
          n151 = xnode ("Register Read")() -> ("Data"=w347:T19)  [unwired: 1 in, 1 out]
          n152 = xnode ("Register Read")() -> ("Data"=w343:sgl)  [unwired: 1 in, 1 out]
          n153 = xnode "Register"() -> ("Data"=w341:u16)  [unwired: 1 in, 1 out]
          n154 = xnode ("Register Read")() -> ("Data"=w342:sgl)  [unwired: 1 in, 1 out]
          n155 = local read "Simultaneous_AI"() -> (w351:sgl[])
          n156 = To Single Precision Float(number=w349) -> (single precision float=w348:sgl)
          n157 = call <instrlib>:"Process.vi"("WaveformAddressSpace in"=w354, "Data"=w350, "Iteration"=w349, "FirstIteration"=w352) -> ("WaveformAddressSpace out"=w353:refnum<class "WaveformAddressSpace.lvclass">, "stop"=w355:bool)  [unwired: 8 in, 2 out]
          n158 = call <userlib>:"FlpLib U32 to SGL Cast.vi"("x"=w341) -> ("y"=w340:sgl)  [unwired: 4 in]
          n159 = Cluster To Array(cluster=w347) -> (array=w344:sgl[])
          n160 = Build Array (concatenate)(w348, w351, w346, w345, w344, w343, w342, w340) -> (w356:sgl[])
          "relativeTimestamp" <- w349
        }
      }
      frame #2 {
        n161 = call <vilib>:"Cleanup.vi"("WaveformAddressSpace in"=w358) -> ()  [unwired: 14 in, 1 out]
      }
    }
  }
  n162 = while "Lowspeed Waveforms" {
    tunnel: w31 -> [w359]
    stop <- FALSE stop-if-true
    n163 = flat-sequence {
      tunnel: [w363] -> w361
      tunnel: w359 -> [w364]
      tunnel: w361 -> [w370]
      tunnel: [w369] -> w360
      tunnel: w360 -> [w387]
      frame #0 {
        n164 = call <vilib>:"Configure.vi"("WaveformAddressSpace in"=w364, "oclk_freq"=u32 40000000, "oclk_mult"=u32 1, "UnderflowMargin"=u32 3 ("y")) -> ("WaveformAddressSpace out"=w363:refnum<class "WaveformAddressSpace.lvclass">)  [unwired: 11 in]
      }
      frame #1 {
        n165 = while {
          shift-right: [w385] -> _
          shift-left: _ -> [w377]
          shift-right: [FALSE] -> _
          shift-left: TRUE -> [w380]
          tunnel: w370 -> [w382]
          tunnel: [w381] -> w369
          i -> [w379]
          stop <- w383 stop-if-true
          n166 = xnode ("Register Read")() -> ("Data"=w375:sgl[])  [unwired: 1 in, 1 out]
          n167 = xnode ("Register Read")() -> ("Data"=w372:sgl)  [unwired: 1 in, 1 out]
          n168 = xnode ("Register Read")() -> ("Data"=w374:sgl)  [unwired: 1 in, 1 out]
          n169 = xnode ("Register Read")() -> ("Data"=w376:T19)  [unwired: 1 in, 1 out]
          n170 = xnode ("Register Read")() -> ("Data"=w371:sgl)  [unwired: 1 in, 1 out]
          n171 = local read "Simultaneous_AI"() -> (w378:sgl[])
          n172 = call <instrlib>:"Process.vi"("WaveformAddressSpace in"=w382, "Data"=w377, "Iteration"=w379, "error in (no error)"=errorcluster {"status"=FALSE, "code"=0, "source"=""} ("injectError1"), "FirstIteration"=w380) -> ("WaveformAddressSpace out"=w381:refnum<class "WaveformAddressSpace.lvclass">, "stop"=w383:bool)  [unwired: 7 in, 2 out]
          n173 = Cluster To Array(cluster=w376) -> (array=w373:sgl[])
          n174 = Build Array (concatenate)(w379, w378, w375, w374, w373, w372, w371) -> (w385:sgl[])
        }
      }
      frame #2 {
        n175 = call <vilib>:"Cleanup.vi"("WaveformAddressSpace in"=w387) -> ()  [unwired: 14 in, 1 out]
      }
    }
  }
  n176 = node-c288(w48) -> ()
  n177 = node-c288(w32) -> ()
  n178 = node-c288(w25) -> ()
